vi "DataLogger.get services.vi"(8 "error in (no error)":errorcluster, 11 "i ref in":refnum<vi>) -> (0 "error out":errorcluster, 3 "i ref out":refnum<vi>)   [LabVIEW 2014, in "DataLogger.lvlib"]
uses:
  DataLogger.lvlib
  CS_Core/BaseProcess/BaseProcess.lvlib
  CS_Core/CSSystem/CoreLib/CoreLib.lvlib
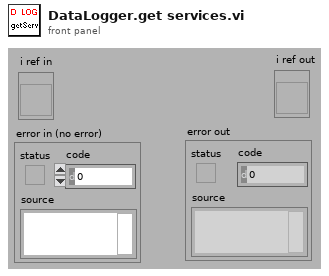
[diagram p1: front panel]
types:
  T1 = typedef "BaseProcess.lvlib/BaseProcess.i attribute.ctl" = cluster{"EventStatus":string, "EventError":i32, "PresetEvtWatchD":i32, "PresetPdcWatchD":i32, "EventTimeout":i32, "PeriodicInterval":i32, "Interface":string[], "Address":string[], "Special":string[], "PeriodicError":i32, "PeriodicStatus":string, "SuperProc":string, "Descriptors":T2[], "CaseRef":refnum<vi>, "PdcRef":refnum<vi>, "Thread Ref":refnum<vi>, "eventErrorID":i32, "eventStatusID":i32, "periodicErrorID":i32, "periodicStatusID":i32, "pdcCtrID":i32}
  T2 = typedef "BaseProcess.lvlib/BaseProcess.descriptor definition.ctl" = cluster{"selector":string, "descriptor":T3}
  T3 = typedef "BaseProcess.lvlib/BaseProcess.descriptor string definition.ctl" = string
  T4 = typedef "DataLogger.lvlib/DataLogger.i attribute.ctl" = cluster{"Service Names":string[], "Path":string[], "Service Alarm Index":i32[], "Service Alarm Limit1":dbl[], "Service Alarm Limit2":dbl[], "Service Alarm Indicator":bool[], "alarmID":i32, "pathID":i32, "SoundDeviceID":i32, "SoundFile":string, "SoundID":i32, "SoundFileID":i32}
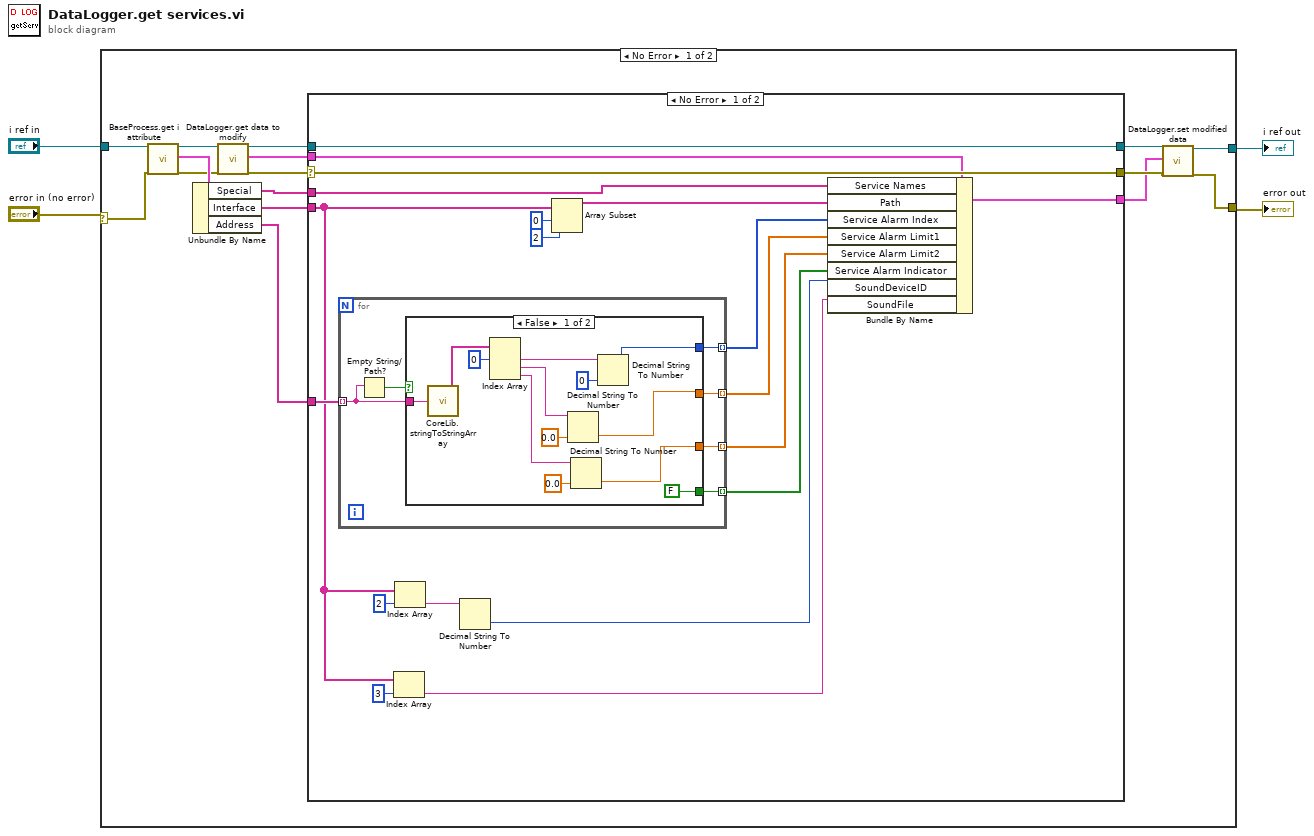
[diagram p0: block diagram]
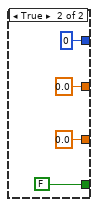
[diagram p2: hidden frame]
diagram:
  n1 = case shown="No Error" "error in (no error)" {
    selector: "error in (no error)" -> [w20 w66]
    tunnel: "i ref in" -> [w19 w67]
    tunnel: [w7 w67] -> w2
    tunnel: [w6 w66] -> w1
    frame No Error {
      n2 = call "BaseProcess.get i attribute.vi"("i ref in"=w19, "error in (no error)"=w20) -> ("i ref out"=w17:refnum<vi>, "i attribute"=w18:T1, "error out"=w15:errorcluster)  [unwired: 15 in]
      n3 = Unbundle By Name(w18) -> ("Special"=w13:string[], "Interface"=w12:string[], "Address"=w5:string[])
      n4 = call "DataLogger.get data to modify.vi"("i ref in"=w17, "error in (no error)"=w15) -> ("i ref out"=w16:refnum<vi>, "i attribute"=w11:T4, "error out"=w14:errorcluster)  [unwired: 14 in, 1 out]
      n5 = case shown="No Error" w14 {
        selector: w14 -> [w38 w65]
        tunnel: w16 -> [w39 w64]
        tunnel: [w39 w64] -> w10
        tunnel: [w38 w65] -> w9
        tunnel: w13 -> [w36 _]
        tunnel: w12 -> [w23 _]
        tunnel: w11 -> [w37 w63]
        tunnel: [w34 w63] -> w8
        tunnel: w5 -> [w35 _]
        frame No Error {
          n6 = for {
            tunnel: w35 -> [w40] mode=indexing
            tunnel: [w45] -> w33 mode=indexing
            tunnel: [w44] -> w32 mode=indexing
            tunnel: [w43] -> w31 mode=indexing
            tunnel: [w42] -> w30 mode=indexing
            n7 = Empty String/Path?(string/path=w40) -> (empty?=w41:bool)
            n8 = case shown="False" w41 {
              tunnel: w40 -> [w57 _]
              tunnel: [w53 0] -> w45
              tunnel: [w50 0.0] -> w44
              tunnel: [w46 0.0] -> w43
              tunnel: [FALSE FALSE] -> w42
              frame False {
                n9 = call "CoreLib.stringToStringArray.vi"("String"=w57) -> ("Array"=w51:string[])
                n10 = Index Array(array=w51, index #1=0 ("index")) -> (element #1=w55:string, element #2=w49:string, element #3=w47:string)  [unwired: 2 in]
                n11 = Decimal String To Number(string=w49, default (0L)=0.0 ("default (0 I32)")) -> (number=w50:dbl)  [unwired: 1 in, 1 out]
                n12 = Decimal String To Number(string=w47, default (0L)=0.0 ("default (0 I32)")) -> (number=w46:dbl)  [unwired: 1 in, 1 out]
                n13 = Decimal String To Number(string=w55, default (0L)=0 ("default (0 I32)")) -> (number=w53:i32)  [unwired: 1 in, 1 out]
              }
              frame True {
              }
            }
          }
          n14 = Index Array(array=w23, index=3) -> (element=w21:string)
          n15 = Index Array(array=w23, index=2) -> (element=w25:string)
          n16 = Decimal String To Number(string=w25) -> (number=w24:i32)  [unwired: 2 in, 1 out]
          n17 = Array Subset(array=w23, index=0, length=2) -> (w27:string[])
          n18 = Bundle By Name(cluster=w37, "Service Names"=w36, "Path"=w27, "Service Alarm Index"=w33, "Service Alarm Limit1"=w32, "Service Alarm Limit2"=w31, "Service Alarm Indicator"=w30, "SoundDeviceID"=w24, "SoundFile"=w21) -> (w34:T4)
        }
        frame Error {
        }
      }
      n19 = call "DataLogger.set modified data.vi"("i ref in"=w10, "i attribute"=w8, "error in (no error)"=w9) -> ("i ref out"=w7:refnum<vi>, "error out"=w6:errorcluster)  [unwired: 15 in]
    }
    frame Error {
    }
  }
  "error out" <- w1
  "i ref out" <- w2
